vi "removeLinesWithPattern.vi"(10 "pattern":string, 11 "text":string) -> (3 "result":string)   [LabVIEW 2023, in "gitTools.lvlib"]
uses:
  gitTools.lvlib
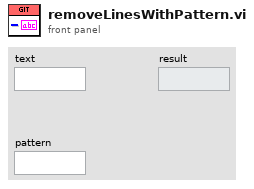
[diagram p1: front panel]
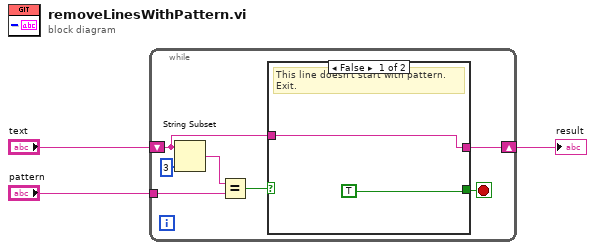
[diagram p0: block diagram]
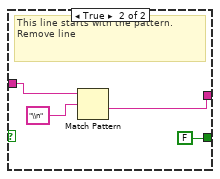
[diagram p2: hidden frame]
diagram:
  n1 = while {
    shift-right: [w10] -> w2
    shift-left: "text" -> [w6]
    tunnel: "pattern" -> [w4]
    stop <- w5 stop-if-true
    n2 = String Subset(string=w6, length (rest)=3 ("length (rest)")) -> (substring=w8:string)  [unwired: 1 in]
    n3 = Equal?(x=w8, y=w4) -> (x = y?=w7:bool)
    n4 = case shown="False" w7 {
      tunnel: [w12 w15] -> w10
      tunnel: w6 -> [w12 w14]
      tunnel: [TRUE FALSE] -> w5
      frame False {
        # "This line doesn't start with pattern.  Exit."
      }
      frame True {
        # "This line starts with the pattern.  Remove line"
        n5 = Match Pattern(string=w14, regular expression="\\n") -> (after substring=w15:string)  [unwired: 1 in, 3 out]
      }
    }
  }
  "result" <- w2
